vi "Array of VData to VCluster.vi"(8 "error in (no error)":errorcluster, 9 "Cluster Name":string, 10 "Array":variant[](array[variant])) -> (0 "error out":errorcluster, 2 "VCluster":variant)   [LabVIEW 2012, in "TD Tools.lvlib"]
uses:
  TD Tools.lvlib
  <userlib>/_OpenG.lib/lvdata/lvdata.llb/Type Descriptor Enumeration__ogtk.ctl
  Custom Type/Type Descriptor.ctl
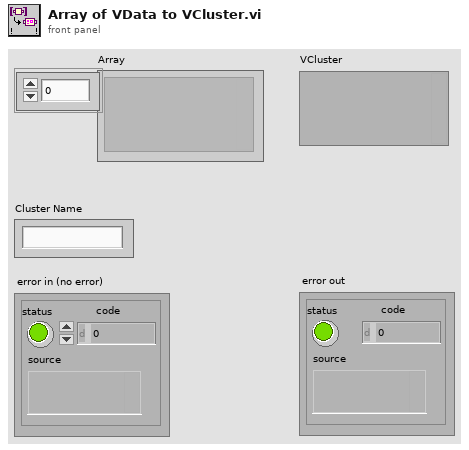
[diagram p1: front panel]
types:
  T1 = typedef "TD Tools.lvlib/Type Descriptor.ctl" = u16[]
  T2 = typedef "Type Descriptor Enumeration__ogtk.ctl" = enum8{"<Null>", "I8", "I16", "I32", "I64", "U8", "U16", "U32", "U64", "SGL", "DBL", "EXT", "CSG", "CDB", "CXT", "0x0F", "0x10", "0x11", "0x12", "0x13", "0x14", "Enum U8", "Enum U16", "Enum U32", "Enum U64", "SGL PQ", "DBL PQ", "EXT PQ", "CSG PQ", "CDB PQ", "CXT PQ", "0x1F", "0x20", "Boolean", "0x22", "0x23", "0x24", "0x25", "0x26", "0x27", "0x28", "0x29", "0x2A", "0x2B", "0x2C", "0x2D", "0x2E", "0x2F", "String", "0x31", "Path", "Pict", "0x34", "0x35", "0x36", "DAQ", "0x38", "0x39", "0x3A", "0x3B", "0x3C", "0x3D", "0x3E", "0x3F", "Array", "0x41", "0x42", "0x43", "0x44", "0x45", "0x46", "0x47", "0x48", "0x49", "0x4A", "0x4B", "0x4C", "0x4D", "0x4E", "0x4F", "Cluster", "0x51", "0x52", "Variant", "Waveform", "0x55", "0x56", "0x57", "0x58", "0x59", "0x5A", "0x5B", "0x5C", "0x5D", "0x5E", "0x5F", "0x60", "0x61", "0x62", "0x63", "0x64", "0x65", "0x66", "0x67", "0x68", "0x69", "0x6A", "0x6B", "0x6C", "0x6D", "0x6E", "0x6F", "Refnum"}
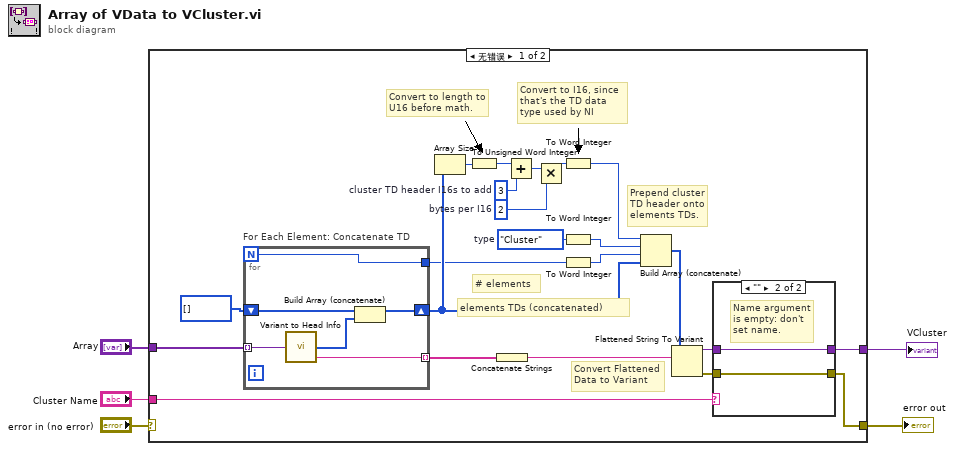
[diagram p0: block diagram]
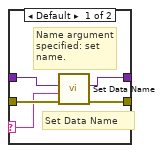
[diagram p2: hidden frame]
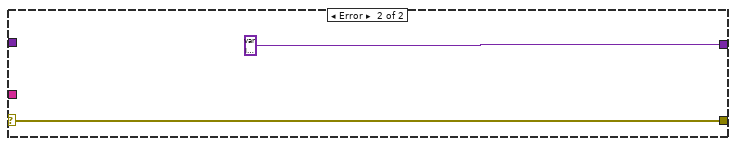
[diagram p3: hidden frame]
diagram:
  n1 = case shown="无错误" "error in (no error)" {
    selector: "error in (no error)" -> [_ w42]
    tunnel: [w15 w42] -> w3
    tunnel: [w17 variant ("Variant")] -> w5
    tunnel: "Array" -> [w19 _]
    tunnel: "Cluster Name" -> [w18 _]
    frame No Error {
      w9 = u16 2  # bytes per I16
      w11 = u16 3  # cluster TD header I16s to add
      w21 = Type_Descriptor_Enumeration__ogtk."Cluster"  # type
      # "Convert Flattened Data to Variant"
      # "elements TDs (concatenated)"
      # "Convert to length to U16 before math."
      # "Convert to I16, since that's the TD data type used by NI"
      # "Prepend cluster TD header onto elements TDs."
      # "# elements"
      n2 = for "For Each Element: Concatenate TD" {
        N -> [w35]
        tunnel: w19 -> [w40] mode=indexing
        tunnel: [w39] -> w27 mode=indexing
        shift-right: [w37] -> w22
        shift-left: T1 [] ("Type Descriptor") -> [w36]
        tunnel: [w35] -> w12
        n3 = call "Variant to Head Info.vi"("Variant"=w40) -> ("Data String"=w39:string, "Type Descriptor"=w38:T1)  [unwired: 2 in, 1 out]
        n4 = Build Array (concatenate)(w36, w38) -> (w37:T1)
      }
      n5 = Array Size(array=w22) -> (size(s)=w24:i32)
      n6 = To Unsigned Word Integer(number=w24) -> (unsigned 16bit integer=w8:u16)
      n7 = Concatenate Strings(w27) -> (w26:string)
      n8 = Add(x=w8, y=w11) -> (x+y=w10:u16)
      n9 = Multiply(x=w10, y=w9) -> (x*y=w7:u16)
      n10 = To Word Integer(number=w7) -> (16bit integer=w23:i16)
      n11 = To Word Integer(number=w21) -> (16bit integer=w13:i16)
      n12 = To Word Integer(number=w12) -> (16bit integer=w20:i16)
      n13 = Build Array (concatenate)(w23, w13, w20, w22) -> (w25:T1)
      n14 = Flattened String To Variant(6:w26, 7:w25) -> (0:w14:errorcluster, 3:w16:variant)  [unwired: 1 in]
      n15 = case shown="\"\"" w18 {
        selector: w18 -> [w30 _]
        tunnel: [w28 w34] -> w17
        tunnel: w16 -> [w29 w34]
        tunnel: [w31 w33] -> w15
        tunnel: w14 -> [w32 w33]
        frame Default {
          # "Set Data Name"
          # "Name argument specified: set name."
          n16 = call "Set Data Name.vi"("错误输入"=w32, "Data Name"=w30, "Data"=w29) -> ("错误输出"=w31:errorcluster, "Renamed Data"=w28:variant)  [unwired: 7 in]
        }
        frame "" {
          # "Name argument is empty: don't set name."
        }
      }
    }
    frame Error {
    }
  }
  "error out" <- w3
  "VCluster" <- w5
